vi "LSMcontroller_v57.vi"() -> ()   [LabVIEW 2015] (continued)
            n3469 = event-data() -> ()  [unwired: 1 in, 6 out]
            n3470 = call "2pparameters.vi"("command"="get") -> ("params out"=w6689:T12)  [unwired: 1 in]
            n3471 = in-place {
              n3472 = in-place-cluster #46(w6689) -> ()  [unwired: 1 out]
              n3473 = local read "auto shutter"() -> (w6691:bool)
              n3474 = in-place-cluster #46("autoshutter"=w6691) -> (w6687:T12)
            }
            n3475 = call "2pparameters.vi"("Params in"=w6687, "command"="set") -> ()  [unwired: 1 out]
          }
          event "auto OD": Value Change {
            n3476 = event-data() -> ()  [unwired: 1 in, 6 out]
            n3477 = call "2pparameters.vi"("command"="get") -> ("params out"=w6694:T12)  [unwired: 1 in]
            n3478 = in-place {
              n3479 = in-place-cluster #47(w6694) -> ()  [unwired: 1 out]
              n3480 = local read "auto OD"() -> (w6696:bool)
              n3481 = in-place-cluster #47("auto OD"=w6696) -> (w6692:T12)
            }
            n3482 = call "2pparameters.vi"("Params in"=w6692, "command"="set") -> ()  [unwired: 1 out]
          }
          event "ODfilt": Value Change {
            n3483 = event-data() -> ("OldVal"=w6697:u16)  [unwired: 1 in, 5 out]
            n3484 = local read "ODfilt"() -> (w6698:u16)
            n3485 = call "2pparameters.vi"("command"="get") -> ("params out"=w6701:T12)  [unwired: 1 in]
            n3486 = call "filterwheelcontrol_nothorlabslib.vi"("Current OD filt"=w6697, "New ODfilt"=w6698) -> ()  [unwired: 1 in]
            n3487 = in-place {
              in-place-border: w6698 -> [w6703]
              n3488 = in-place-cluster #48(w6701) -> ()  [unwired: 1 out]
              n3489 = in-place-cluster #48("ODfilt"=w6703) -> (w6699:T12)
            }
            n3490 = call "2pparameters.vi"("Params in"=w6699, "command"="set") -> ()  [unwired: 1 out]
          }
          event "Exit": Value Change {
            n3491 = event-data() -> ()  [unwired: 1 in, 5 out]
          }
        }
        n3492 = Wait (ms)(milliseconds to wait=u32 50) -> ()  [unwired: 1 out]
      }
      n3493 = while {
        stop <- w75 stop-if-true
        # "Waveform generation"
        n3494 = event shown="[1] \"Add AO wave\": Value Change" {
          selector: _ -> [_ _ _ _ _ _ _ _ _ _ _ _ _ _ _ _ _]
          dyn-events: _ -> [_ _ _ _ _ _ _ _ _ _ _ _ _ _ _ _ _]
          timeout: _ -> [_ _ _ _ _ _ _ _ _ _ _ _ _ _ _ _ _]
          tunnel: [_ _ _ _ _ _ _ _ _ _ _ _ _ _ _ _ w2048] -> w75
          event Timeout {
            n3495 = event-data() -> ()  [unwired: 1 in, 3 out]
          }
          event "Add AO wave": Value Change {
            n3496 = event-data() -> ("NewVal"=w76:bool)  [unwired: 1 in, 5 out]
            n3497 = case shown="True" w76 {
              frame False {
              }
              frame True {
                n3498 = stacked-sequence {
                  frame #0 {
                    n3499 = local read "Measurement"() -> (w77:T5)
                    n3500 = case shown="\"Lifetime (contour)\"" w77 {
                      frame "X-Y-t movie", Default {
                        n3501 = local read "avpp"() -> (w98:i32)
                        n3502 = local read "Angle ref"() -> (w97:dbl)
                        n3503 = local read "ROI Type"() -> (w96:u16)
                        n3504 = local read "xpixels ref"() -> (w93:i32)
                        n3505 = local read "Vx-min ref"() -> (w92:dbl)
                        n3506 = local read "Vx-max ref"() -> (w91:dbl)
                        n3507 = local read "ypixels ref"() -> (w89:i32)
                        n3508 = local read "Vy-min ref"() -> (w90:dbl)
                        n3509 = local read "Vy-max ref"() -> (w86:dbl)
                        n3510 = local read "Sampling rate"() -> (w80:dbl)
                        n3511 = local read "finite samples"() -> (w81:bool)
                        n3512 = local read "continuous"() -> (w84:bool)
                        n3513 = local read "wavdet"() -> (w85:bool)
                        n3514 = local read "# of frames"() -> (w83:i32)
                        n3515 = local read "maxbufferAI"() -> (w82:i32)
                        n3516 = local read "Override AI buffer"() -> (w78:bool)
                        n3517 = call "2pparameters.vi"("command"="get") -> ("params out"=w95:T12)  [unwired: 1 in]
                        n3518 = Bundle By Name(cluster=w95, "type"="X-Y-t movie", "avpp"=w98, "Angle Img"=w97, "Xpixels Img"=w93, "Vx-min Img"=w92, "VX-max Img"=w91, "Ypixels Img"=w89, "Vy-min Img"=w90, "Vy-max Img"=w86, "srate"=w80, "srate Img"=w80, "finite"=w81, "cont"=w84, "wavdet"=w85, "measpoints"=w83, "maxbufferAI"=w82, "Drawing Mode"=w96, "Vz-reset"=0.0, "AIoverride"=w78) -> (w87:T12)
                        n3519 = call "2pparameters.vi"("Params in"=w87, "command"="set") -> ()  [unwired: 1 out]
                      }
                      frame "X-Y-Z stack" {
                        n3520 = call "2pparameters.vi"("command"="get") -> ("params out"=w102:T12)  [unwired: 1 in]
                        n3521 = Bundle By Name(cluster=w102, "type"="X-Y-Z stack") -> (w100:T12)
                        n3522 = call "2pparameters.vi"("Params in"=w100, "command"="set") -> ()  [unwired: 1 out]
                      }
                      frame "Lifetime (scan)" {
                        n3523 = call "2pparameters.vi"("command"="get") -> ("params out"=w107:T12)  [unwired: 1 in]
                        n3524 = Bundle By Name(cluster=w107, "type"="Lifetime (scan)") -> (w105:T12)
                        n3525 = call "2pparameters.vi"("Params in"=w105, "command"="set") -> ()  [unwired: 1 out]
                      }
                      frame "Lifetime (contour)" {
                        n3526 = local read "Vy-min draw"() -> (w117:dbl)
                        n3527 = local read "Vy-max draw"() -> (w116:dbl)
                        n3528 = local read "Vx-min draw"() -> (w119:dbl)
                        n3529 = local read "Vx-max draw"() -> (w118:dbl)
                        n3530 = local read "xpixels ref"() -> (w115:i32)
                        n3531 = local read "ypixels ref"() -> (w114:i32)
                        n3532 = local read "ROI Type"() -> (w113:u16)
                        n3533 = local read "srateAODOtt"() -> (w124:dbl)
                        n3534 = local read "# of frames"() -> (w129:i32)
                        n3535 = local read "refreshtime"() -> (w121:dbl)
                        n3536 = local read "Pel"() -> (w112:dbl)
                        n3537 = local read "bin"() -> (w127:dbl)
                        n3538 = local read "Override AI buffer"() -> (w110:bool)
                        n3539 = local read "finite samples"() -> (w136:bool)
                        n3540 = local read "srateAODOtt"() -> (w123:dbl)
                        n3541 = local read "srateAODOtt"() -> (w130:dbl)
                        n3542 = local read "continuous"() -> (w135:bool)
                        n3543 = local read "Angle ref"() -> (w120:dbl)
                        n3544 = local read "wavdet"() -> (w137:bool)
                        n3545 = local read "Vx-ref"() -> (w132:dbl)
                        n3546 = local read "Vy-ref"() -> (w134:dbl)
                        n3547 = local read "avpp"() -> (w133:i32)
                        n3548 = call "tt_timeandsamples.vi"("bin"=w127, "refreshtime"=w121, "srateAODOtt"=w124, "tot#ofsamples"=w129) -> ("refreshrate"=w125:dbl, "refreshbuffer"=w126:i32, "timetracecycles"=w131:i32)  [unwired: 5 in]
                        n3549 = local read "bin"() -> (w128:dbl)
                        n3550 = call "2pparameters.vi"("command"="get") -> ("params out"=w140:T12)  [unwired: 1 in]
                        n3551 = Bundle By Name(cluster=w140, "Drawing Mode"=w113, "measpoints"=w129, "tt_cycles"=w131, "refreshbuffer"=w126, "refreshrate"=w125, "Vx-ref"=w132, "Vy-ref"=w134, "srate"=w123, "finite"=w136, "cont"=w135, "wavdet"=w137, "avpp"=w133, "srateAODO"=w130, "bufferAI"=w126, "bin"=w128, "Angle Img"=w120, "Vxminref"=w119, "Vxmaxref"=w118, "Vyminref"=w117, "Vymaxref"=w116, "Xpixels Img"=w115, "Ypixels Img"=w114, "Pel"=w112, "Vz-reset"=0.0, "AIoverride"=w110, "type"="Lifetime (contour)") -> (w138:T12)
                        n3552 = Reciprocal(x=w125) -> (1/x=w122:dbl)
                        n3553 = local write "refreshtime"(w122) -> ()
                        n3554 = call "2pparameters.vi"("Params in"=w138, "command"="set") -> ()  [unwired: 1 out]
                      }
                      frame "X-Y-Z-t movie" {
                      }
                      frame "linescan" {
                      }
                      frame "Timetrace" {
                        n3555 = local read "Vy-min draw"() -> (w150:dbl)
                        n3556 = local read "Vy-max draw"() -> (w149:dbl)
                        n3557 = local read "Vx-min draw"() -> (w152:dbl)
                        n3558 = local read "Vx-max draw"() -> (w151:dbl)
                        n3559 = local read "xpixels ref"() -> (w148:i32)
                        n3560 = local read "ypixels ref"() -> (w147:i32)
                        n3561 = local read "ROI Type"() -> (w146:u16)
                        n3562 = local read "srateAODOtt"() -> (w157:dbl)
                        n3563 = local read "# of frames"() -> (w162:i32)
                        n3564 = local read "refreshtime"() -> (w154:dbl)
                        n3565 = local read "Pel"() -> (w145:dbl)
                        n3566 = local read "bin"() -> (w160:dbl)
                        n3567 = local read "Override AI buffer"() -> (w143:bool)
                        n3568 = local read "finite samples"() -> (w169:bool)
                        n3569 = local read "srateAODOtt"() -> (w156:dbl)
                        n3570 = local read "srateAODOtt"() -> (w163:dbl)
                        n3571 = local read "continuous"() -> (w168:bool)
                        n3572 = local read "Angle ref"() -> (w153:dbl)
                        n3573 = local read "wavdet"() -> (w170:bool)
                        n3574 = local read "Vx-ref"() -> (w165:dbl)
                        n3575 = local read "Vy-ref"() -> (w167:dbl)
                        n3576 = local read "avpp"() -> (w166:i32)
                        n3577 = call "tt_timeandsamples.vi"("bin"=w160, "refreshtime"=w154, "srateAODOtt"=w157, "tot#ofsamples"=w162) -> ("refreshrate"=w158:dbl, "refreshbuffer"=w159:i32, "timetracecycles"=w164:i32)  [unwired: 5 in]
                        n3578 = local read "bin"() -> (w161:dbl)
                        n3579 = call "2pparameters.vi"("command"="get") -> ("params out"=w173:T12)  [unwired: 1 in]
                        n3580 = Bundle By Name(cluster=w173, "Drawing Mode"=w146, "measpoints"=w162, "tt_cycles"=w164, "refreshbuffer"=w159, "refreshrate"=w158, "Vx-ref"=w165, "Vy-ref"=w167, "srate"=w156, "finite"=w169, "cont"=w168, "wavdet"=w170, "avpp"=w166, "srateAODO"=w163, "bufferAI"=w159, "bin"=w161, "Angle Img"=w153, "Vxminref"=w152, "Vxmaxref"=w151, "Vyminref"=w150, "Vymaxref"=w149, "Xpixels Img"=w148, "Ypixels Img"=w147, "Pel"=w145, "Vz-reset"=0.0, "AIoverride"=w143, "type"="Timetrace") -> (w171:T12)
                        n3581 = Reciprocal(x=w158) -> (1/x=w155:dbl)
                        n3582 = local write "refreshtime"(w155) -> ()
                        n3583 = call "2pparameters.vi"("Params in"=w171, "command"="set") -> ()  [unwired: 1 out]
                      }
                      frame "Lifetime (point)" {
                      }
                    }
                  }
                  frame #1 {
                    w176 = FALSE ("wavdet")
                    n3584 = call "2pparameters.vi"("command"="get") -> ("params out"=w180:T12)  [unwired: 1 in]
                    n3585 = Bundle By Name(cluster=w180, "finite"=w176, "cont"=w176, "wavdet"=TRUE) -> (w177:T12)
                    n3586 = call "2pparameters.vi"("Params in"=w177, "command"="set") -> ()  [unwired: 1 out]
                  }
                  frame #2 {
                    # "change active waveform numbers array"
                    n3587 = local read "AO channels"() -> (w187:u32)
                    n3588 = call "2pparameters.vi"("command"="get") -> ("params out"=w185:T12)  [unwired: 1 in]
                    n3589 = in-place {
                      in-place-border: w187 -> [w191]
                      in-place-border: [w188] -> w182
                      n3590 = in-place-cluster #49(w185) -> ("aAO"=w190:u32[])
                      n3591 = call "add channel to active arrayv2.vi"("line array in"=w190, "line to add"=w191) -> ("line array out"=w189:u32[], "addition"=w188:bool)  [unwired: 1 out]
                      n3592 = in-place-cluster #49("aAO"=w189) -> (w183:T12)
                    }
                    n3593 = local write "addAO"(w182) -> ()
                    n3594 = call "2pparameters.vi"("Params in"=w183, "command"="set") -> ()  [unwired: 1 out]
                  }
                  frame #3 {
                    # "update GUI"
                    n3595 = local read "addAO"() -> (w192:bool)
                    n3596 = case shown="True" w192 {
                      frame False {
                      }
                      frame True {
                        n3597 = call "Used AO lines.vi"() -> ("used AO names"=w196:string[], "used AO lines"=w198:tag[])  [unwired: 2 in]
                        n3598 = control-ref of="Analog Lines Plot"() -> (w197:refnum<vi>)
                        n3599 = control-ref of="Digital Lines Plot"() -> (w195:refnum<vi>)
                        n3600 = call "Used DO lines.vi"() -> ("used DO names"=w194:string[], "used DO lines"=w193:tag[])  [unwired: 2 in]
                        n3601 = local write "Analog Used Lines"(w198) -> ()
                        n3602 = local write "Analog Used Names"(w196) -> ()
                        n3603 = local write "Digital Used Lines"(w193) -> ()
                        n3604 = local write "Digital Used Names"(w194) -> ()
                        n3605 = call "prepDOWaveplot.vi"("DigitalGraph in"=w195, "used DO names"=w194) -> ()  [unwired: 1 in]
                        n3606 = call "prepAOWaveplot.vi"("WaveformGraph in"=w197, "Analog Used Names"=w196) -> ()  [unwired: 1 in]
                      }
                    }
                  }
                  frame #4 {
                    n3607 = local read "addAO"() -> (w199:bool)
                    n3608 = case shown="True" w199 {
                      frame False {
                      }
                      frame True {
                        # "add parameters\nto parameter array"
                        n3609 = local read "Build analog waveform tabs"() -> (w200:enum32{"Square", "Triangle", "Matlab"})
                        n3610 = case shown="\"Square\", Default" w200 {
                          frame "Square", Default {
                            w213 = 0.0 ("Offset (V)")
                            n3611 = local read "Meastab"() -> (w202:enum32{"X-Y Image", "Linescan", "Timetrace"})
                            n3612 = call "waveformparamsv2.vi"("command"="get") -> ("Params out"=w211:T16)  [unwired: 4 in, 2 out]
                            n3613 = Unbundle By Name(w211) -> ("AO parameters"=w208:T17)
                            n3614 = case shown="\"Timetrace\"" w202 {
                              tunnel: [w224 w225] -> w201
                              frame "X-Y Image", Default {
                                n3615 = local read "Sampling rate"() -> (w224:dbl)
                              }
                              frame "Timetrace" {
                                n3616 = local read "srateAODOtt"() -> (w225:dbl)
                              }
                            }
                            n3617 = local read "Start amplitude (V)"() -> (w221:dbl)
                            n3618 = local read "phase shift (ms)"() -> (w214:dbl)
                            n3619 = local read "Step size (V)"() -> (w219:dbl)
                            n3620 = local read "Baseline (V)"() -> (w220:dbl)
                            n3621 = local read "Period (ms)"() -> (w217:dbl)
                            n3622 = local read "padding value"() -> (w204:dbl)
                            n3623 = local read "Repeats"() -> (w223:dbl)
                            n3624 = local read "DC (%)"() -> (w218:dbl)
                            n3625 = local read "Cycles"() -> (w222:dbl)
                            n3626 = local read "Pulses"() -> (w215:dbl)
                            n3627 = Index Array(array=w208, index=0) -> (element=w209:T18)
                            n3628 = Bundle By Name(cluster=w209, "AOtab"=0.0 ("Repeats"), "Repeats"=w223, "Cycles"=w222, "Start amplitude (V)"=w221, "Baseline (V)"=w220, "Step size (V)"=w219, "DC (%)"=w218, "Sampling frequency (Hz)"=w201, "Period (ms)"=w217, "Offset (V)"=w213, "Amplitude (V)"=w213, "Frequency"=w213, "Tri Repeats"=w213, "phase shift (ms)"=w214, "Pulses"=w215, "Matlab wave file"=path "", "padding value"=w204) -> (w206:T18)
                            n3629 = Build Array(w206) -> (w205:T17)
                            n3630 = call "waveformparamsv2.vi"("command"="add AO", "add AO"=w205) -> ()  [unwired: 3 in, 3 out]
                          }
                          frame "Matlab" {
                            w231 = 0.0 ("Repeats")
                            n3631 = local read "Meastab"() -> (w227:enum32{"X-Y Image", "Linescan", "Timetrace"})
                            n3632 = call "waveformparamsv2.vi"("command"="get") -> ("Params out"=w238:T16)  [unwired: 4 in, 2 out]
                            n3633 = Unbundle By Name(w238) -> ("AO parameters"=w235:T17)
                            n3634 = case shown="\"Timetrace\"" w227 {
                              tunnel: [w241 w242] -> w226
                              frame "X-Y Image", Default {
                                n3635 = local read "Sampling rate"() -> (w241:dbl)
                              }
                              frame "Timetrace" {
                                n3636 = local read "srateAODOtt"() -> (w242:dbl)
                              }
                            }
                            n3637 = local read "Matlab waveform path"() -> (w228:path)
                            n3638 = local read "Matlab padding value"() -> (w230:dbl)
                            n3639 = Index Array(array=w235, index=0) -> (element=w236:T18)
                            n3640 = call "matlabwfexistsdialogue.vi"("Matlab waveform path"=w228) -> ("mtalab waveform path out"=w229:path)
                            n3641 = Bundle By Name(cluster=w236, "AOtab"=2.0 ("Repeats"), "Repeats"=w231, "Cycles"=w231, "Start amplitude (V)"=w231, "Baseline (V)"=w231, "Step size (V)"=w231, "DC (%)"=w231, "Sampling frequency (Hz)"=w226, "Period (ms)"=w231, "Offset (V)"=w231, "Amplitude (V)"=w231, "Frequency"=w231, "Tri Repeats"=w231, "phase shift (ms)"=w231, "Pulses"=w231, "Matlab wave file"=w229, "padding value"=w230) -> (w233:T18)
                            n3642 = Build Array(w233) -> (w232:T17)
                            n3643 = call "waveformparamsv2.vi"("command"="add AO", "add AO"=w232) -> ()  [unwired: 3 in, 3 out]
                          }
                          frame "Triangle" {
                            w248 = 0.0 ("Offset (V)")
                            n3644 = local read "Meastab"() -> (w244:enum32{"X-Y Image", "Linescan", "Timetrace"})
                            n3645 = call "waveformparamsv2.vi"("command"="get") -> ("Params out"=w260:T16)  [unwired: 4 in, 2 out]
                            n3646 = Unbundle By Name(w260) -> ("AO parameters"=w257:T17)
                            n3647 = case shown="\"Timetrace\"" w244 {
                              tunnel: [w262 w263] -> w243
                              frame "X-Y Image", Default {
                                n3648 = local read "Sampling rate"() -> (w262:dbl)
                              }
                              frame "Timetrace" {
                                n3649 = local read "srateAODOtt"() -> (w263:dbl)
                              }
                            }
                            n3650 = local read "Tri padding value"() -> (w246:dbl)
                            n3651 = local read "Amplitude (V)"() -> (w251:dbl)
                            n3652 = local read "Tri Phase (s)"() -> (w247:dbl)
                            n3653 = local read "Tri Repeats"() -> (w249:dbl)
                            n3654 = local read "Frequency"() -> (w250:dbl)
                            n3655 = local read "Offset (V)"() -> (w252:dbl)
                            n3656 = Index Array(array=w257, index=0) -> (element=w258:T18)
                            n3657 = Bundle By Name(cluster=w258, "AOtab"=1.0 ("Repeats"), "Repeats"=w248, "Cycles"=w248, "Start amplitude (V)"=w248, "Baseline (V)"=w248, "Step size (V)"=w248, "DC (%)"=w248, "Sampling frequency (Hz)"=w243, "Period (ms)"=w248, "Offset (V)"=w252, "Amplitude (V)"=w251, "Frequency"=w250, "Tri Repeats"=w249, "phase shift (ms)"=w248, "Pulses"=w248, "Matlab wave file"=path "", "Tri phase"=w247, "padding value"=w246) -> (w255:T18)
                            n3658 = Build Array(w255) -> (w254:T17)
                            n3659 = call "waveformparamsv2.vi"("command"="add AO", "add AO"=w254) -> ()  [unwired: 3 in, 3 out]
                          }
                        }
                      }
                    }
                  }
                  frame #5 {
                    n3660 = local read "addAO"() -> (w264:bool)
                    n3661 = case shown="True" w264 {
                      frame False {
                      }
                      frame True {
                        # "add waveform to waveform array; correct waveform lengths and plot"
                        n3662 = local read "Meastab"() -> (w268:enum32{"X-Y Image", "Linescan", "Timetrace"})
                        n3663 = local read "Build analog waveform tabs"() -> (w278:enum32{"Square", "Triangle", "Matlab"})
                        n3664 = case shown="\"Timetrace\"" w268 {
                          tunnel: [w286 w287] -> w267
                          frame "X-Y Image", Default {
                            n3665 = local read "Sampling rate"() -> (w286:dbl)
                          }
                          frame "Timetrace" {
                            n3666 = local read "srateAODOtt"() -> (w287:dbl)
                          }
                        }
                        n3667 = call "waveformparamsv2.vi"("command"="get last AO") -> ("last AO"=w280:T18)  [unwired: 4 in, 2 out]
                        n3668 = case shown="\"Matlab\"" w278 {
                          tunnel: w280 -> [w290 w292 w294]
                          tunnel: [w289 w291 w293] -> w279
                          frame "Square", Default {
                            n3669 = call "generateRampedSquareWave_fromAOparameters.vi"("AO params"=w290) -> ("Waveform"=w289:waveform(dbl))  [unwired: 1 out]
                          }
                          frame "Triangle" {
                            n3670 = call "generateTriWave_fromAOparameters.vi"("AO params"=w292) -> ("Waveform"=w291:waveform(dbl))  [unwired: 1 out]
                          }
                          frame "Matlab" {
                            n3671 = call "matlabAOwffromparam.vi"("Cluster"=w294) -> ("Waveform"=w293:waveform(dbl))  [unwired: 1 out]
                          }
                        }
                        n3672 = property on="refwf" class="Ring (strict)"() -> ("RingText.Text"=w271:string)  [unwired: 2 in, 2 out]
                        n3673 = call "waveformsAObuffer.vi"("command"="get") -> ("AO wf out"=w284:waveform(dbl)[])  [unwired: 1 in]
                        n3674 = Build Array (concatenate)(w284, w279) -> (w281:waveform(dbl)[])
                        n3675 = call "waveformsDObuffer.vi"("command"="get") -> ("DO wf out"=w276:digitalwaveform[])  [unwired: 1 in]
                        n3676 = call "correctwaveformsizetemp.vi"("new sampling frequency (Hz)"=w267, "start"=FALSE, "reference waveforms to"=w271, "Analog waveforms in"=w281, "stop"=FALSE, "Digital waveforms in"=w276) -> ("analog wf out"=w274:waveform(dbl)[], "Digital wf out"=w272:digitalwaveform[], "measpoints"=w269:i32)
                        n3677 = local write "Analog Lines Plot"(w274) -> ()
                        n3678 = call "GetNumCamFramesv2.vi"("Digital Waveform Graph"=w272) -> ("Numeric"=w273:i32)  [unwired: 10 in]
                        n3679 = local write "Digital Lines Plot"(w272) -> ()
                        n3680 = call "waveformsAObuffer.vi"("AO wf in"=w274, "command"="set") -> ()  [unwired: 1 out]
                        n3681 = call "waveformsDObuffer.vi"("DO wf in"=w272, "command"="set") -> ()  [unwired: 1 out]
                        n3682 = local write "Total Camera Frames"(w273) -> ()
                        n3683 = local read "wavdet"() -> (w270:bool)
                        n3684 = case shown="True" w270 {
                          tunnel: w269 -> [_ w288]
                          frame False {
                          }
                          frame True {
                            n3685 = local write "# of frames"(w288) -> ()
                          }
                        }
                      }
                    }
                  }
                  frame #6 {
                    w295 = FALSE ("addAO")
                    # "set signaling boolean to false"
                    n3686 = local read "finite samples"() -> (w296:bool)
                    n3687 = local read "continuous"() -> (w297:bool)
                    n3688 = local read "wavdet"() -> (w298:bool)
                    n3689 = call "2pparameters.vi"("command"="get") -> ("params out"=w301:T12)  [unwired: 1 in]
                    n3690 = Bundle By Name(cluster=w301, "finite"=w296, "cont"=w297, "wavdet"=w298) -> (w299:T12)
                    n3691 = local write "addAO"(w295) -> ()
                    n3692 = property on="Add AO wave" class="Bool (strict)"("Val(Sgnl)"=w295) -> ()  [unwired: 2 in, 2 out]
                    n3693 = call "2pparameters.vi"("Params in"=w299, "command"="set") -> ()  [unwired: 1 out]
                  }
                }
              }
            }
          }
          event "AO channels": Value Change {
            n3694 = event-data() -> ()  [unwired: 1 in, 6 out]
            n3695 = local read "AO channels"() -> (w303:u32)
            n3696 = call "2pparameters.vi"("command"="get") -> ("params out"=w305:T12)  [unwired: 1 in]
            n3697 = Unbundle By Name(w305) -> ("aAO"=w304:u32[])
            n3698 = Search 1D Array(1D array=w304, element=w303) -> (index of element=w307:i32)  [unwired: 1 in]
            n3699 = Equal?(x=w307, y=-1.0) -> (x = y?=w308:bool)
            n3700 = case shown="False" w308 {
              tunnel: w307 -> [w310 _]
              frame False {
                n3701 = call "waveformparamsv2.vi"("command"="get") -> ("Params out"=w317:T16)  [unwired: 4 in, 2 out]
                n3702 = Unbundle By Name(w317) -> ("AO parameters"=w316:T17)
                n3703 = Index Array(array=w316, index=w310) -> (element=w333:T18)
                n3704 = Unbundle By Name(w333) -> ("AOtab"=w314:dbl, "Repeats"=w332:dbl, "Cycles"=w331:dbl, "Start amplitude (V)"=w330:dbl, "Baseline (V)"=w329:dbl, "Step size (V)"=w328:dbl, "DC (%)"=w327:dbl, "Sampling frequency (Hz)"=w326:dbl, "Period (ms)"=w325:dbl, "Offset (V)"=w324:dbl, "Amplitude (V)"=w323:dbl, "Frequency"=w322:dbl, "Tri Repeats"=w321:dbl, "phase shift (ms)"=w320:dbl, "Pulses"=w319:dbl, "Tri phase"=w315:dbl, "padding value"=w311:dbl, "Matlab wave file"=w312:path)
                n3705 = To Unsigned Long Integer(number=w314) -> (unsigned 32bit integer=w313:u32)
                n3706 = local write "Build analog waveform tabs"(w313) -> ()
                n3707 = local write "Matlab waveform path"(w312) -> ()
                n3708 = local write "phase shift (ms)"(w320) -> ()
                n3709 = local write "Repeats"(w332) -> ()
                n3710 = local write "Cycles"(w331) -> ()
                n3711 = local write "Amplitude (V)"(w323) -> ()
                n3712 = local write "Matlab padding value"(w311) -> ()
                n3713 = local write "Tri padding value"(w311) -> ()
                n3714 = local write "Start amplitude (V)"(w330) -> ()
                n3715 = local write "Tri Phase (s)"(w315) -> ()
                n3716 = local write "Period (ms)"(w325) -> ()
                n3717 = local write "Tri Repeats"(w321) -> ()
                n3718 = local write "Offset (V)"(w324) -> ()
                n3719 = local write "Frequency"(w322) -> ()
                n3720 = local write "Pulses"(w319) -> ()
                n3721 = local write "padding value"(w311) -> ()
                n3722 = local write "Sampling rate \ncurrent wf"(w326) -> ()
                n3723 = local write "Baseline (V)"(w329) -> ()
                n3724 = local write "Step size (V)"(w328) -> ()
                n3725 = local write "DC (%)"(w327) -> ()
                "Numeric" <- w310
              }
              frame True {
              }
            }
          }
          event "Rem AO wave": Value Change {
            n3726 = event-data() -> ("NewVal"=w334:bool)  [unwired: 1 in, 5 out]
            n3727 = case shown="True" w334 {
              frame False {
              }
              frame True {
                n3728 = stacked-sequence {
                  seq-local: [_ _ w440 _ _ _ _] -> [_ _ _ _ w460 w463 _]
                  frame #0 {
                    n3729 = local read "Measurement"() -> (w335:T5)
                    n3730 = case shown="\"X-Y-t movie\", Default" w335 {
                      frame "X-Y-t movie", Default {
                        n3731 = local read "avpp"() -> (w356:i32)
                        n3732 = local read "Angle ref"() -> (w355:dbl)
                        n3733 = local read "ROI Type"() -> (w354:u16)
                        n3734 = local read "xpixels ref"() -> (w351:i32)
                        n3735 = local read "Vx-min ref"() -> (w350:dbl)
                        n3736 = local read "Vx-max ref"() -> (w349:dbl)
                        n3737 = local read "ypixels ref"() -> (w347:i32)
                        n3738 = local read "Vy-min ref"() -> (w348:dbl)
                        n3739 = local read "Vy-max ref"() -> (w344:dbl)
                        n3740 = local read "Sampling rate"() -> (w338:dbl)
                        n3741 = local read "finite samples"() -> (w339:bool)
                        n3742 = local read "continuous"() -> (w342:bool)
                        n3743 = local read "wavdet"() -> (w343:bool)
                        n3744 = local read "# of frames"() -> (w341:i32)
                        n3745 = local read "maxbufferAI"() -> (w340:i32)
                        n3746 = local read "Override AI buffer"() -> (w336:bool)
                        n3747 = call "2pparameters.vi"("command"="get") -> ("params out"=w353:T12)  [unwired: 1 in]
                        n3748 = Bundle By Name(cluster=w353, "type"="X-Y-t movie", "avpp"=w356, "Angle Img"=w355, "Xpixels Img"=w351, "Vx-min Img"=w350, "VX-max Img"=w349, "Ypixels Img"=w347, "Vy-min Img"=w348, "Vy-max Img"=w344, "srate"=w338, "srate Img"=w338, "finite"=w339, "cont"=w342, "wavdet"=w343, "measpoints"=w341, "maxbufferAI"=w340, "Drawing Mode"=w354, "Vz-reset"=0.0, "AIoverride"=w336) -> (w345:T12)
                        n3749 = call "2pparameters.vi"("Params in"=w345, "command"="set") -> ()  [unwired: 1 out]
                      }
                      frame "X-Y-Z stack" {
                        n3750 = call "2pparameters.vi"("command"="get") -> ("params out"=w360:T12)  [unwired: 1 in]
                        n3751 = Bundle By Name(cluster=w360, "type"="X-Y-Z stack") -> (w358:T12)
                        n3752 = call "2pparameters.vi"("Params in"=w358, "command"="set") -> ()  [unwired: 1 out]
                      }
                      frame "Lifetime (scan)" {
                        n3753 = call "2pparameters.vi"("command"="get") -> ("params out"=w365:T12)  [unwired: 1 in]
                        n3754 = Bundle By Name(cluster=w365, "type"="Lifetime (scan)") -> (w363:T12)
                        n3755 = call "2pparameters.vi"("Params in"=w363, "command"="set") -> ()  [unwired: 1 out]
                      }
                      frame "Lifetime (contour)" {
                        n3756 = local read "Vy-min draw"() -> (w375:dbl)
                        n3757 = local read "Vy-max draw"() -> (w374:dbl)
                        n3758 = local read "Vx-min draw"() -> (w377:dbl)
                        n3759 = local read "Vx-max draw"() -> (w376:dbl)
                        n3760 = local read "xpixels ref"() -> (w373:i32)
                        n3761 = local read "ypixels ref"() -> (w372:i32)
                        n3762 = local read "ROI Type"() -> (w371:u16)
                        n3763 = local read "srateAODOtt"() -> (w382:dbl)
                        n3764 = local read "# of frames"() -> (w387:i32)
                        n3765 = local read "refreshtime"() -> (w379:dbl)
                        n3766 = local read "Pel"() -> (w370:dbl)
                        n3767 = local read "bin"() -> (w385:dbl)
                        n3768 = local read "Override AI buffer"() -> (w368:bool)
                        n3769 = local read "finite samples"() -> (w394:bool)
                        n3770 = local read "srateAODOtt"() -> (w381:dbl)
                        n3771 = local read "srateAODOtt"() -> (w388:dbl)
                        n3772 = local read "continuous"() -> (w393:bool)
                        n3773 = local read "Angle ref"() -> (w378:dbl)
                        n3774 = local read "wavdet"() -> (w395:bool)
                        n3775 = local read "Vx-ref"() -> (w390:dbl)
                        n3776 = local read "Vy-ref"() -> (w392:dbl)
                        n3777 = local read "avpp"() -> (w391:i32)
                        n3778 = call "tt_timeandsamples.vi"("bin"=w385, "refreshtime"=w379, "srateAODOtt"=w382, "tot#ofsamples"=w387) -> ("refreshrate"=w383:dbl, "refreshbuffer"=w384:i32, "timetracecycles"=w389:i32)  [unwired: 5 in]
                        n3779 = local read "bin"() -> (w386:dbl)
                        n3780 = call "2pparameters.vi"("command"="get") -> ("params out"=w398:T12)  [unwired: 1 in]
                        n3781 = Bundle By Name(cluster=w398, "Drawing Mode"=w371, "measpoints"=w387, "tt_cycles"=w389, "refreshbuffer"=w384, "refreshrate"=w383, "Vx-ref"=w390, "Vy-ref"=w392, "srate"=w381, "finite"=w394, "cont"=w393, "wavdet"=w395, "avpp"=w391, "srateAODO"=w388, "bufferAI"=w384, "bin"=w386, "Angle Img"=w378, "Vxminref"=w377, "Vxmaxref"=w376, "Vyminref"=w375, "Vymaxref"=w374, "Xpixels Img"=w373, "Ypixels Img"=w372, "Pel"=w370, "Vz-reset"=0.0, "AIoverride"=w368, "type"="Lifetime (contour)") -> (w396:T12)
                        n3782 = Reciprocal(x=w383) -> (1/x=w380:dbl)
                        n3783 = local write "refreshtime"(w380) -> ()
                        n3784 = call "2pparameters.vi"("Params in"=w396, "command"="set") -> ()  [unwired: 1 out]
                      }
                      frame "X-Y-Z-t movie" {
                      }
                      frame "linescan" {
                      }
                      frame "Timetrace" {
                        n3785 = local read "Vy-min draw"() -> (w408:dbl)
                        n3786 = local read "Vy-max draw"() -> (w407:dbl)
                        n3787 = local read "Vx-min draw"() -> (w410:dbl)
                        n3788 = local read "Vx-max draw"() -> (w409:dbl)
                        n3789 = local read "xpixels ref"() -> (w406:i32)
                        n3790 = local read "ypixels ref"() -> (w405:i32)
                        n3791 = local read "ROI Type"() -> (w404:u16)
                        n3792 = local read "srateAODOtt"() -> (w415:dbl)
                        n3793 = local read "# of frames"() -> (w420:i32)
                        n3794 = local read "refreshtime"() -> (w412:dbl)
                        n3795 = local read "Pel"() -> (w403:dbl)
                        n3796 = local read "bin"() -> (w418:dbl)
                        n3797 = local read "Override AI buffer"() -> (w401:bool)
                        n3798 = local read "finite samples"() -> (w427:bool)
                        n3799 = local read "srateAODOtt"() -> (w414:dbl)
                        n3800 = local read "srateAODOtt"() -> (w421:dbl)
                        n3801 = local read "continuous"() -> (w426:bool)
                        n3802 = local read "Angle ref"() -> (w411:dbl)
                        n3803 = local read "wavdet"() -> (w428:bool)
                        n3804 = local read "Vx-ref"() -> (w423:dbl)
                        n3805 = local read "Vy-ref"() -> (w425:dbl)
                        n3806 = local read "avpp"() -> (w424:i32)
                        n3807 = call "tt_timeandsamples.vi"("bin"=w418, "refreshtime"=w412, "srateAODOtt"=w415, "tot#ofsamples"=w420) -> ("refreshrate"=w416:dbl, "refreshbuffer"=w417:i32, "timetracecycles"=w422:i32)  [unwired: 5 in]
                        n3808 = local read "bin"() -> (w419:dbl)
                        n3809 = call "2pparameters.vi"("command"="get") -> ("params out"=w431:T12)  [unwired: 1 in]
                        n3810 = Bundle By Name(cluster=w431, "Drawing Mode"=w404, "measpoints"=w420, "tt_cycles"=w422, "refreshbuffer"=w417, "refreshrate"=w416, "Vx-ref"=w423, "Vy-ref"=w425, "srate"=w414, "finite"=w427, "cont"=w426, "wavdet"=w428, "avpp"=w424, "srateAODO"=w421, "bufferAI"=w417, "bin"=w419, "Angle Img"=w411, "Vxminref"=w410, "Vxmaxref"=w409, "Vyminref"=w408, "Vymaxref"=w407, "Xpixels Img"=w406, "Ypixels Img"=w405, "Pel"=w403, "Vz-reset"=0.0, "AIoverride"=w401, "type"="Timetrace") -> (w429:T12)
                        n3811 = Reciprocal(x=w416) -> (1/x=w413:dbl)
                        n3812 = local write "refreshtime"(w413) -> ()
                        n3813 = call "2pparameters.vi"("Params in"=w429, "command"="set") -> ()  [unwired: 1 out]
                      }
                      frame "Lifetime (point)" {
                      }
                    }
                  }
                  frame #1 {
                    w434 = FALSE ("wavdet")
                    n3814 = call "2pparameters.vi"("command"="get") -> ("params out"=w438:T12)  [unwired: 1 in]
                    n3815 = Bundle By Name(cluster=w438, "finite"=w434, "cont"=w434, "wavdet"=TRUE) -> (w435:T12)
                    n3816 = call "2pparameters.vi"("Params in"=w435, "command"="set") -> ()  [unwired: 1 out]
                  }
                  frame #2 {
                    # "remove channel from numbers array"
                    n3817 = local read "AO channels"() -> (w445:u32)
                    n3818 = call "2pparameters.vi"("command"="get") -> ("params out"=w443:T12)  [unwired: 1 in]
                    n3819 = in-place {
                      in-place-border: w445 -> [w451]
                      in-place-border: [w448] -> w446
                      in-place-border: [w447] -> w440
                      n3820 = in-place-cluster #50(w443) -> ("aAO"=w450:u32[])
                      n3821 = call "remove channel from active arrayv2.vi"("line array in"=w450, "line to remove"=w451) -> ("line array out"=w449:u32[], "removal"=w448:bool, "index"=w447:i32)
                      n3822 = in-place-cluster #50("aAO"=w449) -> (w441:T12)
                    }
                    n3823 = local write "remAO"(w446) -> ()
                    n3824 = call "2pparameters.vi"("Params in"=w441, "command"="set") -> ()  [unwired: 1 out]
                  }
                  frame #3 {
                    n3825 = local read "remAO"() -> (w452:bool)
                    n3826 = case shown="True" w452 {
                      frame False {
                      }
                      frame True {
                        n3827 = call "Used AO lines.vi"() -> ("used AO names"=w456:string[], "used AO lines"=w458:tag[])  [unwired: 2 in]
                        n3828 = control-ref of="Analog Lines Plot"() -> (w457:refnum<vi>)
                        n3829 = control-ref of="Digital Lines Plot"() -> (w455:refnum<vi>)
                        n3830 = call "Used DO lines.vi"() -> ("used DO names"=w454:string[], "used DO lines"=w453:tag[])  [unwired: 2 in]
                        n3831 = local write "Analog Used Lines"(w458) -> ()
                        n3832 = local write "Analog Used Names"(w456) -> ()
                        n3833 = local write "Digital Used Lines"(w453) -> ()
                        n3834 = local write "Digital Used Names"(w454) -> ()
                        n3835 = call "prepDOWaveplot.vi"("DigitalGraph in"=w455, "used DO names"=w454) -> ()  [unwired: 1 in]
                        n3836 = call "prepAOWaveplot.vi"("WaveformGraph in"=w457, "Analog Used Names"=w456) -> ()  [unwired: 1 in]
                      }
                    }
                  }
                  frame #4 {
                    n3837 = local read "remAO"() -> (w459:bool)
                    n3838 = case shown="True" w459 {
                      tunnel: w460 -> [_ w461]
                      frame False {
                      }
                      frame True {
                        n3839 = call "waveformparamsv2.vi"("command"="rem AO", "index"=w461) -> ()  [unwired: 3 in, 3 out]
                      }
                    }
                  }
                  frame #5 {
                    n3840 = local read "remAO"() -> (w464:bool)
                    n3841 = case shown="True" w464 {
                      tunnel: w463 -> [_ w483]
                      frame False {
                      }
                      frame True {
                        n3842 = local read "Meastab"() -> (w468:enum32{"X-Y Image", "Linescan", "Timetrace"})
                        n3843 = property on="refwf" class="Ring (strict)"() -> ("RingText.Text"=w471:string)  [unwired: 2 in, 2 out]
                        n3844 = case shown="\"Timetrace\"" w468 {
                          tunnel: [w484 w485] -> w467
                          frame "X-Y Image", Default {
                            n3845 = local read "Sampling rate"() -> (w484:dbl)
                          }
                          frame "Timetrace" {
                            n3846 = local read "srateAODOtt"() -> (w485:dbl)
                          }
                        }
                        n3847 = call "waveformsAObuffer.vi"("command"="get") -> ("AO wf out"=w480:waveform(dbl)[])  [unwired: 1 in]
                        n3848 = call "waveformsDObuffer.vi"("command"="get") -> ("DO wf out"=w477:digitalwaveform[])  [unwired: 1 in]
                        n3849 = Delete From Array(array=w480, length=1, index=w483) -> (array with subset deleted=w472:waveform(dbl)[])  [unwired: 1 out]
                        n3850 = call "correctwaveformsizetemp.vi"("new sampling frequency (Hz)"=w467, "start"=FALSE, "reference waveforms to"=w471, "Analog waveforms in"=w472, "stop"=FALSE, "Digital waveforms in"=w477) -> ("analog wf out"=w475:waveform(dbl)[], "Digital wf out"=w473:digitalwaveform[], "measpoints"=w469:i32)
                        n3851 = local write "Analog Lines Plot"(w475) -> ()
                        n3852 = call "GetNumCamFramesv2.vi"("Digital Waveform Graph"=w473) -> ("Numeric"=w474:i32)  [unwired: 10 in]
                        n3853 = local write "Digital Lines Plot"(w473) -> ()
                        n3854 = call "waveformsAObuffer.vi"("AO wf in"=w475, "command"="set") -> ()  [unwired: 1 out]
                        n3855 = call "waveformsDObuffer.vi"("DO wf in"=w473, "command"="set") -> ()  [unwired: 1 out]
                        n3856 = local read "wavdet"() -> (w470:bool)
                        n3857 = local write "Total Camera Frames"(w474) -> ()
                        n3858 = case shown="True" w470 {
                          tunnel: w469 -> [_ w486]
                          frame False {
                          }
                          frame True {
                            n3859 = local write "# of frames"(w486) -> ()
                          }
                        }
                      }
                    }
                  }
                  frame #6 {
                    w487 = FALSE ("remAO")
                    n3860 = local read "finite samples"() -> (w488:bool)
                    n3861 = local read "continuous"() -> (w489:bool)
                    n3862 = local read "wavdet"() -> (w490:bool)
                    n3863 = call "2pparameters.vi"("command"="get") -> ("params out"=w493:T12)  [unwired: 1 in]
                    n3864 = Bundle By Name(cluster=w493, "finite"=w488, "cont"=w489, "wavdet"=w490) -> (w491:T12)
                    n3865 = local write "remAO"(w487) -> ()
                    n3866 = property on="Rem AO wave" class="Bool (strict)"("Val(Sgnl)"=w487) -> ()  [unwired: 2 in, 2 out]
                    n3867 = call "2pparameters.vi"("Params in"=w491, "command"="set") -> ()  [unwired: 1 out]
                  }
                }
              }
            }
          }
          event "Add DO wave": Value Change {
            n3868 = event-data() -> ("NewVal"=w495:bool)  [unwired: 1 in, 5 out]
            n3869 = case shown="True" w495 {
              frame False {
              }
              frame True {
                n3870 = stacked-sequence {
                  seq-local: [_ _ _ _ _ w655 _ _] -> [_ _ _ _ _ _ w670 _]
                  frame #0 {
                    n3871 = local read "Measurement"() -> (w496:T5)
                    n3872 = case shown="\"X-Y-t movie\", Default" w496 {
                      frame "X-Y-t movie", Default {
                        n3873 = local read "avpp"() -> (w517:i32)
                        n3874 = local read "Angle ref"() -> (w516:dbl)
                        n3875 = local read "ROI Type"() -> (w515:u16)
                        n3876 = local read "xpixels ref"() -> (w512:i32)
                        n3877 = local read "Vx-min ref"() -> (w511:dbl)
                        n3878 = local read "Vx-max ref"() -> (w510:dbl)
                        n3879 = local read "ypixels ref"() -> (w508:i32)
                        n3880 = local read "Vy-min ref"() -> (w509:dbl)
                        n3881 = local read "Vy-max ref"() -> (w505:dbl)
                        n3882 = local read "Sampling rate"() -> (w499:dbl)
                        n3883 = local read "finite samples"() -> (w500:bool)
                        n3884 = local read "continuous"() -> (w503:bool)
                        n3885 = local read "wavdet"() -> (w504:bool)
                        n3886 = local read "# of frames"() -> (w502:i32)
                        n3887 = local read "maxbufferAI"() -> (w501:i32)
                        n3888 = local read "Override AI buffer"() -> (w497:bool)
                        n3889 = call "2pparameters.vi"("command"="get") -> ("params out"=w514:T12)  [unwired: 1 in]
                        n3890 = Bundle By Name(cluster=w514, "type"="X-Y-t movie", "avpp"=w517, "Angle Img"=w516, "Xpixels Img"=w512, "Vx-min Img"=w511, "VX-max Img"=w510, "Ypixels Img"=w508, "Vy-min Img"=w509, "Vy-max Img"=w505, "srate"=w499, "srate Img"=w499, "finite"=w500, "cont"=w503, "wavdet"=w504, "measpoints"=w502, "maxbufferAI"=w501, "Drawing Mode"=w515, "Vz-reset"=0.0, "AIoverride"=w497) -> (w506:T12)
                        n3891 = call "2pparameters.vi"("Params in"=w506, "command"="set") -> ()  [unwired: 1 out]
                      }
                      frame "X-Y-Z stack" {
                        n3892 = call "2pparameters.vi"("command"="get") -> ("params out"=w521:T12)  [unwired: 1 in]
                        n3893 = Bundle By Name(cluster=w521, "type"="X-Y-Z stack") -> (w519:T12)
                        n3894 = call "2pparameters.vi"("Params in"=w519, "command"="set") -> ()  [unwired: 1 out]
                      }
                      frame "Lifetime (scan)" {
                        n3895 = call "2pparameters.vi"("command"="get") -> ("params out"=w526:T12)  [unwired: 1 in]
                        n3896 = Bundle By Name(cluster=w526, "type"="Lifetime (scan)") -> (w524:T12)
                        n3897 = call "2pparameters.vi"("Params in"=w524, "command"="set") -> ()  [unwired: 1 out]
                      }
                      frame "Lifetime (contour)" {
                        n3898 = local read "Vy-min draw"() -> (w536:dbl)
                        n3899 = local read "Vy-max draw"() -> (w535:dbl)
                        n3900 = local read "Vx-min draw"() -> (w538:dbl)
                        n3901 = local read "Vx-max draw"() -> (w537:dbl)
                        n3902 = local read "xpixels ref"() -> (w534:i32)
                        n3903 = local read "ypixels ref"() -> (w533:i32)
                        n3904 = local read "ROI Type"() -> (w532:u16)
                        n3905 = local read "srateAODOtt"() -> (w543:dbl)
                        n3906 = local read "# of frames"() -> (w548:i32)
                        n3907 = local read "refreshtime"() -> (w540:dbl)
                        n3908 = local read "Pel"() -> (w531:dbl)
                        n3909 = local read "bin"() -> (w546:dbl)
                        n3910 = local read "Override AI buffer"() -> (w529:bool)
                        n3911 = local read "finite samples"() -> (w555:bool)
                        n3912 = local read "srateAODOtt"() -> (w542:dbl)
                        n3913 = local read "srateAODOtt"() -> (w549:dbl)
                        n3914 = local read "continuous"() -> (w554:bool)
                        n3915 = local read "Angle ref"() -> (w539:dbl)
                        n3916 = local read "wavdet"() -> (w556:bool)
                        n3917 = local read "Vx-ref"() -> (w551:dbl)
                        n3918 = local read "Vy-ref"() -> (w553:dbl)
                        n3919 = local read "avpp"() -> (w552:i32)
                        n3920 = call "tt_timeandsamples.vi"("bin"=w546, "refreshtime"=w540, "srateAODOtt"=w543, "tot#ofsamples"=w548) -> ("refreshrate"=w544:dbl, "refreshbuffer"=w545:i32, "timetracecycles"=w550:i32)  [unwired: 5 in]
                        n3921 = local read "bin"() -> (w547:dbl)
                        n3922 = call "2pparameters.vi"("command"="get") -> ("params out"=w559:T12)  [unwired: 1 in]
                        n3923 = Bundle By Name(cluster=w559, "Drawing Mode"=w532, "measpoints"=w548, "tt_cycles"=w550, "refreshbuffer"=w545, "refreshrate"=w544, "Vx-ref"=w551, "Vy-ref"=w553, "srate"=w542, "finite"=w555, "cont"=w554, "wavdet"=w556, "avpp"=w552, "srateAODO"=w549, "bufferAI"=w545, "bin"=w547, "Angle Img"=w539, "Vxminref"=w538, "Vxmaxref"=w537, "Vyminref"=w536, "Vymaxref"=w535, "Xpixels Img"=w534, "Ypixels Img"=w533, "Pel"=w531, "Vz-reset"=0.0, "AIoverride"=w529, "type"="Lifetime (contour)") -> (w557:T12)
                        n3924 = Reciprocal(x=w544) -> (1/x=w541:dbl)
                        n3925 = local write "refreshtime"(w541) -> ()
                        n3926 = call "2pparameters.vi"("Params in"=w557, "command"="set") -> ()  [unwired: 1 out]
                      }
                      frame "X-Y-Z-t movie" {
                      }
                      frame "linescan" {
                      }
                      frame "Timetrace" {
                        n3927 = local read "Vy-min draw"() -> (w569:dbl)
                        n3928 = local read "Vy-max draw"() -> (w568:dbl)
                        n3929 = local read "Vx-min draw"() -> (w571:dbl)
                        n3930 = local read "Vx-max draw"() -> (w570:dbl)
                        n3931 = local read "xpixels ref"() -> (w567:i32)
                        n3932 = local read "ypixels ref"() -> (w566:i32)
                        n3933 = local read "ROI Type"() -> (w565:u16)
                        n3934 = local read "srateAODOtt"() -> (w576:dbl)
                        n3935 = local read "# of frames"() -> (w581:i32)
                        n3936 = local read "refreshtime"() -> (w573:dbl)
                        n3937 = local read "Pel"() -> (w564:dbl)
                        n3938 = local read "bin"() -> (w579:dbl)
                        n3939 = local read "Override AI buffer"() -> (w562:bool)
                        n3940 = local read "finite samples"() -> (w588:bool)
                        n3941 = local read "srateAODOtt"() -> (w575:dbl)
                        n3942 = local read "srateAODOtt"() -> (w582:dbl)
                        n3943 = local read "continuous"() -> (w587:bool)
                        n3944 = local read "Angle ref"() -> (w572:dbl)
                        n3945 = local read "wavdet"() -> (w589:bool)
                        n3946 = local read "Vx-ref"() -> (w584:dbl)
                        n3947 = local read "Vy-ref"() -> (w586:dbl)
                        n3948 = local read "avpp"() -> (w585:i32)
                        n3949 = call "tt_timeandsamples.vi"("bin"=w579, "refreshtime"=w573, "srateAODOtt"=w576, "tot#ofsamples"=w581) -> ("refreshrate"=w577:dbl, "refreshbuffer"=w578:i32, "timetracecycles"=w583:i32)  [unwired: 5 in]
                        n3950 = local read "bin"() -> (w580:dbl)
                        n3951 = call "2pparameters.vi"("command"="get") -> ("params out"=w592:T12)  [unwired: 1 in]
                        n3952 = Bundle By Name(cluster=w592, "Drawing Mode"=w565, "measpoints"=w581, "tt_cycles"=w583, "refreshbuffer"=w578, "refreshrate"=w577, "Vx-ref"=w584, "Vy-ref"=w586, "srate"=w575, "finite"=w588, "cont"=w587, "wavdet"=w589, "avpp"=w585, "srateAODO"=w582, "bufferAI"=w578, "bin"=w580, "Angle Img"=w572, "Vxminref"=w571, "Vxmaxref"=w570, "Vyminref"=w569, "Vymaxref"=w568, "Xpixels Img"=w567, "Ypixels Img"=w566, "Pel"=w564, "Vz-reset"=0.0, "AIoverride"=w562, "type"="Timetrace") -> (w590:T12)
                        n3953 = Reciprocal(x=w577) -> (1/x=w574:dbl)
                        n3954 = local write "refreshtime"(w574) -> ()
                        n3955 = call "2pparameters.vi"("Params in"=w590, "command"="set") -> ()  [unwired: 1 out]
                      }
                      frame "Lifetime (point)" {
                      }
                    }
                  }
                  frame #1 {
                    w595 = FALSE ("wavdet")
                    n3956 = call "2pparameters.vi"("command"="get") -> ("params out"=w599:T12)  [unwired: 1 in]
                    n3957 = Bundle By Name(cluster=w599, "finite"=w595, "cont"=w595, "wavdet"=TRUE) -> (w596:T12)
                    n3958 = call "2pparameters.vi"("Params in"=w596, "command"="set") -> ()  [unwired: 1 out]
                  }
                  frame #2 {
                    n3959 = local read "DO channels"() -> (w606:u16)
                    n3960 = call "2pparameters.vi"("command"="get") -> ("params out"=w604:T12)  [unwired: 1 in]
                    n3961 = in-place {
                      in-place-border: w606 -> [w610]
                      in-place-border: [w607] -> w601
                      n3962 = in-place-cluster #51(w604) -> ("aDO"=w609:u32[])
                      n3963 = call "add channel to active arrayv2.vi"("line array in"=w609, "line to add"=w610) -> ("line array out"=w608:u32[], "addition"=w607:bool)  [unwired: 1 out]
                      n3964 = in-place-cluster #51("aDO"=w608) -> (w602:T12)
                    }
                    n3965 = local write "addDO"(w601) -> ()
                    n3966 = call "2pparameters.vi"("Params in"=w602, "command"="set") -> ()  [unwired: 1 out]
                  }
                  frame #3 {
                    n3967 = local read "addDO"() -> (w611:bool)
                    n3968 = case shown="True" w611 {
                      frame False {
                      }
                      frame True {
                        n3969 = call "Used AO lines.vi"() -> ("used AO names"=w615:string[], "used AO lines"=w617:tag[])  [unwired: 2 in]
                        n3970 = control-ref of="Analog Lines Plot"() -> (w616:refnum<vi>)
                        n3971 = control-ref of="Digital Lines Plot"() -> (w614:refnum<vi>)
                        n3972 = call "Used DO lines.vi"() -> ("used DO names"=w613:string[], "used DO lines"=w612:tag[])  [unwired: 2 in]
                        n3973 = local write "Analog Used Lines"(w617) -> ()
                        n3974 = local write "Analog Used Names"(w615) -> ()
                        n3975 = local write "Digital Used Lines"(w612) -> ()
                        n3976 = local write "Digital Used Names"(w613) -> ()
                        n3977 = call "prepDOWaveplot.vi"("DigitalGraph in"=w614, "used DO names"=w613) -> ()  [unwired: 1 in]
                        n3978 = call "prepAOWaveplot.vi"("WaveformGraph in"=w616, "Analog Used Names"=w615) -> ()  [unwired: 1 in]
                      }
                    }
                  }
                  frame #4 {
                    n3979 = local read "addDO"() -> (w618:bool)
                    n3980 = case shown="True" w618 {
                      frame False {
                      }
                      frame True {
                        n3981 = local read "Build digital waveform tabs"() -> (w619:enum32{"Simple", "Matlab"})
                        n3982 = case shown="\"Matlab\"" w619 {
                          frame "Simple", Default {
                            n3983 = local read "Meastab"() -> (w621:enum32{"X-Y Image", "Linescan", "Timetrace"})
                            n3984 = call "waveformparamsv2.vi"("command"="get") -> ("Params out"=w635:T16)  [unwired: 4 in, 2 out]
                            n3985 = case shown="\"Timetrace\"" w621 {
                              tunnel: [w637 w638] -> w620
                              frame "X-Y Image", Default {
                                n3986 = local read "Sampling rate"() -> (w637:dbl)
                              }
                              frame "Timetrace" {
                                n3987 = local read "srateAODOtt"() -> (w638:dbl)
                              }
                            }
                            n3988 = Unbundle By Name(w635) -> ("DO parameters"=w633:T19)
                            n3989 = local read "Digital padding value"() -> (w624:dbl)
                            n3990 = local read "Digital time offset (s)"() -> (w625:dbl)
                            n3991 = local read "Digital phase (s)"() -> (w627:dbl)
                            n3992 = local read "Digital Freq (Hz)"() -> (w626:dbl)
                            n3993 = local read "Digital DC (%)"() -> (w628:dbl)
                            n3994 = Index Array(array=w633, index=0) -> (element=w632:T20)
                            n3995 = Bundle By Name(cluster=w632, "Digital DC (%)"=w628, "Digital phase"=w627, "Digital Freq (Hz)"=w626, "Sampling frequency (Hz)"=w620, "Digital time offset (s)"=w625, "padding value"=w624, "matlab wave file"=path "", "DOtab"=0.0) -> (w630:T20)
                            n3996 = Build Array(w630) -> (w629:T19)
                            n3997 = call "waveformparamsv2.vi"("command"="add DO", "add DO"=w629) -> ()  [unwired: 3 in, 3 out]
                          }
                          frame "Matlab" {
                            w642 = 0.0 ("DOtab")
                            n3998 = local read "Meastab"() -> (w640:enum32{"X-Y Image", "Linescan", "Timetrace"})
                            n3999 = call "waveformparamsv2.vi"("command"="get") -> ("Params out"=w651:T16)  [unwired: 4 in, 2 out]
                            n4000 = case shown="\"Timetrace\"" w640 {
                              tunnel: [w653 w654] -> w639
                              frame "X-Y Image", Default {
                                n4001 = local read "Sampling rate"() -> (w653:dbl)
                              }
                              frame "Timetrace" {
                                n4002 = local read "srateAODOtt"() -> (w654:dbl)
                              }
                            }
                            n4003 = Unbundle By Name(w651) -> ("DO parameters"=w649:T19)
                            n4004 = local read "Matlab waveform path DO"() -> (w641:path)
                            n4005 = local read "Matlab padding value DO"() -> (w644:dbl)
                            n4006 = Index Array(array=w649, index=0) -> (element=w648:T20)
                            n4007 = Bundle By Name(cluster=w648, "Digital DC (%)"=w642, "Digital phase"=w642, "Digital Freq (Hz)"=w642, "Sampling frequency (Hz)"=w639, "Digital time offset (s)"=w642, "padding value"=w644, "matlab wave file"=w641, "DOtab"=1.0) -> (w646:T20)
                            n4008 = Build Array(w646) -> (w645:T19)
                            n4009 = call "waveformparamsv2.vi"("command"="add DO", "add DO"=w645) -> ()  [unwired: 3 in, 3 out]
                          }
                        }
                      }
                    }
                  }
                  frame #5 {
                    n4010 = local read "addDO"() -> (w656:bool)
                    n4011 = case shown="True" w656 {
                      tunnel: [_ w657] -> w655
                      frame False {
                      }
                      frame True {
                        n4012 = property on="refwf" class="Ring (strict)"() -> ("RingText.Text"=w662:string)  [unwired: 2 in, 2 out]
                        n4013 = call "waveformsDObuffer.vi"("command"="get") -> ("DO wf out"=w661:digitalwaveform[])  [unwired: 1 in]
                        n4014 = call "waveformsAObuffer.vi"("command"="get") -> ("AO wf out"=w659:waveform(dbl)[])  [unwired: 1 in]
                        n4015 = call "referfencesize.vi"("Digital waveforms in"=w661, "Analog waveforms in"=w659, "reference waveforms to"=w662) -> ("number of samples"=w657:i32)  [unwired: 2 in]
                      }
                    }
                  }
                  frame #6 {
                    n4016 = local read "Build digital waveform tabs"() -> (w673:enum32{"Simple", "Matlab"})
                    n4017 = call "waveformparamsv2.vi"("command"="get last DO") -> ("last DO"=w672:T20)  [unwired: 4 in, 2 out]
                    n4018 = local read "Meastab"() -> (w666:enum32{"X-Y Image", "Linescan", "Timetrace"})
                    n4019 = call "waveformsDObuffer.vi"("command"="get") -> ("DO wf out"=w671:digitalwaveform[])  [unwired: 1 in]
                    n4020 = case shown="\"Simple\", Default" w673 {
                      tunnel: w672 -> [w690 w692]
                      tunnel: w670 -> [w689 _]
                      tunnel: [w688 w691] -> w669
                      frame "Simple", Default {
                        n4021 = call "simple digital from wf params.vi"("waveform params"=w690, "number of samples"=w689) -> ("digital waveform"=w688:digitalwaveform)
                      }
                      frame "Matlab" {
                        n4022 = call "matlabDOwffromparam.vi"("waveform params"=w692) -> ("digital waveform"=w691:digitalwaveform)
                      }
                    }
                    n4023 = property on="refwf" class="Ring (strict)"() -> ("RingText.Text"=w676:string)  [unwired: 2 in, 2 out]
                    n4024 = case shown="\"Timetrace\"" w666 {
                      tunnel: [w685 w686] -> w665
